vi "DIALOG_Mass Compile_ACAF.vi"(8 "error in (no error)":errorcluster) -> (0 "error out":errorcluster, 3 "user event out":refnum<user-event>)   [LabVIEW 2023]
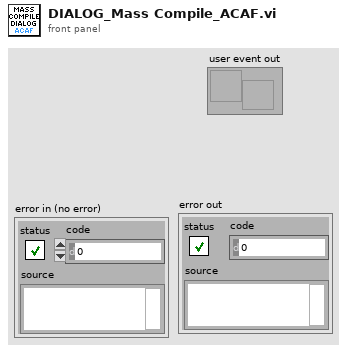
[diagram p1: front panel]
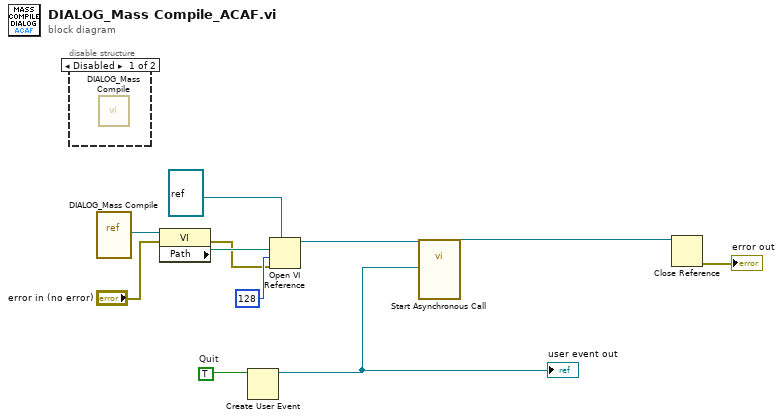
[diagram p0: block diagram]
diagram:
  w4 = TRUE  # Quit
  n1 = disable-structure shown="Disabled" {
    frame Disabled {
      n2 = call "DIALOG_Mass Compile.vi"() -> ()  [unwired: 12 in]
    }
    frame Enabled {
    }
  }
  n3 = vi-ref "DIALOG_Mass Compile.vi"() -> (w8:refnum<vi>)
  n4 = property class="VI"(reference=w8, error in="error in (no error)") -> (error out=w5:errorcluster, "Path"=w7:path)  [unwired: 1 out]
  n5 = Create User Event(user event datatype=w4) -> (user event=w1:refnum<user-event>)  [unwired: 1 in, 1 out]
  "user event out" <- w1
  n6 = Open VI Reference(type specifier VI Refnum (for type only)=refnum<vi> refnum ("reference"), vi path=w7, options=128, error in (no error)=w5) -> (vi reference=w3:refnum<vi>)  [unwired: 2 in, 1 out]
  n7 = call-by-ref "Start Asynchronous Call"(reference=w3, "Quit UE"=w1) -> (reference out=w2:refnum<vi>)  [unwired: 12 in, 1 out]
  n8 = Close Reference(reference=w2) -> (error out=→"error out":errorcluster)  [unwired: 1 in]
